vi "IR_UDP.vi"() -> ()   [LabVIEW 2015]
doc: "The myRIO Project template acquires acceleration data from the onboard accelerometer and displays the changes of acceleration values in a waveform chart."
uses:
  <vilib>/myRIO/Instrument Drivers/Utilities/Utilities.lvlib
  <vilib>/NIOSC/NI_OSC.lvlib
  <vilib>/NIOSC/Create Int32 Argument.vi
  <vilib>/NIOSC/Create Message_Single Arg.vi
  <vilib>/ptbypt/NI_PtbyPt.lvlib
  <vilib>/myRIO/Express VI/Onboard IO/AI/AI Express VI.xnode
  <vilib>/myRIO/Instrument Drivers/Onboard IO/AI/vis/Read.vi
  <vilib>/myRIO/Instrument Drivers/Onboard IO/AI/AI.lvlib
  <vilib>/myRIO/Common/Instrument Driver Framework/Utilities/typedefs/Analog Scaling Constants.ctl
  <vilib>/myRIO/Common/Instrument Driver Framework/Utilities/typedefs/Analog Scaling Constants List.ctl
  <vilib>/myRIO/Common/Instrument Driver Framework/myRIO v1.0/AI/typedefs/AI Channels Enum.ctl
  <vilib>/myRIO/Common/Instrument Driver Framework/myRIO v1.0/AI/typedefs/AI Channels List.ctl
  <vilib>/myRIO/Common/Instrument Driver Framework/Utilities/typedefs/Generic FPGA Reference.ctl
  <vilib>/myRIO/Common/Instrument Driver Framework/Utilities/typedefs/myRIO v1.0 Reference.ctl
  <vilib>/myRIO/Common/Instrument Driver Framework/Utilities/typedefs/Hardware Version Enum.ctl
  <vilib>/myRIO/Common/Instrument Driver Framework/Utilities/typedefs/myRIO Generic Hardware Reference.ctl
  <vilib>/myRIO/Instrument Drivers/Onboard IO/AI/typedefs/AI Reference.ctl
  <vilib>/myRIO/Instrument Drivers/Onboard IO/AI/vis/myRIO AI Open.xnode
  <vilib>/myRIO/Common/Instrument Driver Framework/Utilities/vis/Is FPGA Ref Available.vi
  <vilib>/myRIO/Common/Instrument Driver Framework/myRIO v1.0/AI/vis/myRIO v1.1 Open AI.vi
  <vilib>/userdefined/High Color/nirio_resource_hc.ctl
panel:
  out "numeric 2":dbl format="%_3g"
  in  "Koffset [cm] 2":dbl
  in  "Kscale [cm-V] 2":dbl=27.5
  out "Vo [V] 2":dbl format="%.2f"
  out "Range [cm] 2":dbl(knob) scale=0.0..10.0
  out "error out":errorcluster
  in  "Stop":bool
  # "Overview: The myRIO Project template acquires acceleration data from the onboard accelerometer and displays the changes of acceleration values in a waveform chart.\nInstructions:\n1. Check the myRIO target IP address in the project and make sure the target IP address is correct. \n2. Run this VI."
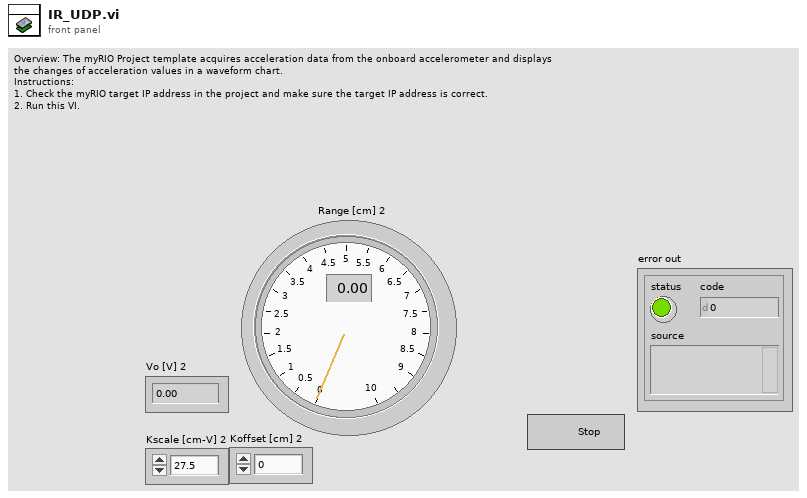
[diagram p1: front panel]
types:
  T1 = typedef "AI.lvlib/AI Reference.ctl" = cluster{"myRIO Reference":T2, "AI Channels List":T6, "AI Scaling Constants List":T8}
  T2 = typedef "myRIO Generic Hardware Reference.ctl" = cluster{"myRIO Model":T3, "myRIO Hardware Reference":T4}
  T3 = typedef "Hardware Version Enum.ctl" = enum16{"Unknown", "myRIO-1900", "myRIO-1950", "roboRIO"}
  T4 = typedef "myRIO v1.0 Reference.ctl" = cluster{"Generic FPGA Reference":T5, "Allow multiple opens":bool}
  T5 = typedef "Generic FPGA Reference.ctl" = refnum<k20>
  T6 = typedef "AI Channels List.ctl" = T7[]
  T7 = typedef "AI Channels Enum.ctl" = enum16{"Not Connected", "AudioIn/Left", "AudioIn/Right", "C/AI0", "C/AI1", "A/AI0", "A/AI1", "A/AI2", "A/AI3", "B/AI0", "B/AI1", "B/AI2", "B/AI3", "AI/AI0", "AI/AI1", "AI/AI2", "AI/AI3"}
  T8 = typedef "Analog Scaling Constants List.ctl" = T9[]
  T9 = typedef "Analog Scaling Constants.ctl" = cluster{"LSB Weight (Volts)":dbl, "Offset (Volts)":dbl, "Signed?":bool}
  T10 = typedef "nirio_resource_hc.ctl" = tag
  T11 = typedef "NI_OSC.lvlib/Argument.ctl" = cluster{"argument":string, "type tag":string}
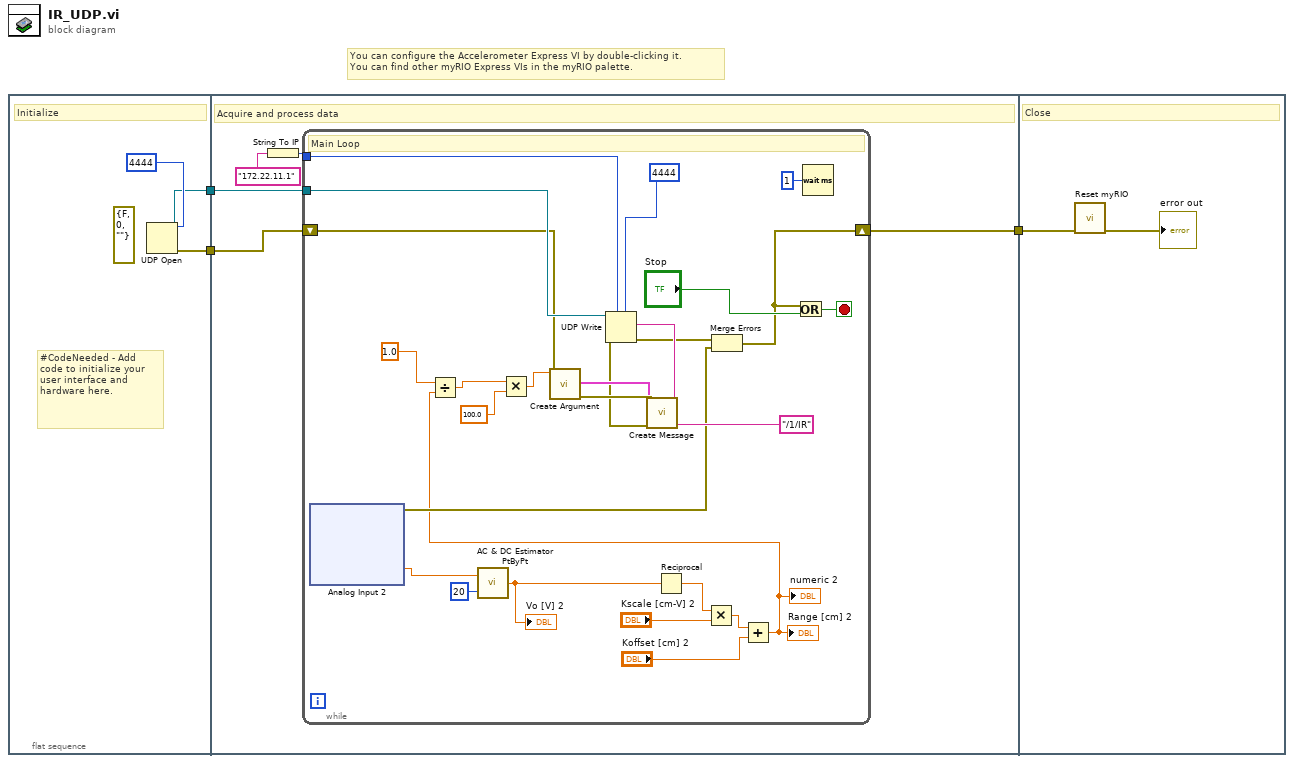
[diagram p0: block diagram]
diagram:
  # "You can configure the Accelerometer Express VI by double-clicking it.\nYou can find other myRIO Express VIs in the myRIO palette."
  n1 = flat-sequence {
    tunnel: [w4] -> w3
    tunnel: [w5] -> w2
    tunnel: w3 -> [w11]
    tunnel: w2 -> [w10]
    tunnel: [w7] -> w1
    tunnel: w1 -> [w76]
    frame #0 {
      (unwired) errorcluster {"status"=FALSE, "code"=0, "source"=""} ("error in (no error)")
      # "#CodeNeeded - Add code to initialize your user interface and hardware here."
      # "Initialize"
      n2 = UDP Open(11:u16 4444 ("port")) -> (port=w5:refnum<k16>, 0:w4:errorcluster)  [unwired: 4 in, 1 out]
    }
    frame #1 {
      # "Acquire and process data"
      n3 = String To IP(1:"172.22.11.1" ("data")) -> (0:w8:u32)
      n4 = while {
        shift-right: [w19] -> w7
        shift-left: w11 -> [w31]
        tunnel: w10 -> [w35]
        tunnel: w8 -> [w33]
        stop <- w37 stop-if-true
        # "Main Loop"
        n5 = xnode "Analog Input 2"() -> ("B/AI0 (Pin 3)"=w20:dbl, "error out"=w17:errorcluster)  [unwired: 1 in]
        n6 = call <vilib>:"AC & DC Estimator PtByPt.vi"("signal"=w20, "sample length"=20) -> ("DC estimate (V)"=w24:dbl)  [unwired: 1 in, 2 out]
        "Vo [V] 2" <- w24
        n7 = Reciprocal(x=w24) -> (1/x=w26:dbl)
        n8 = Multiply(x=w26, y="Kscale [cm-V] 2") -> (x*y=w21:dbl)
        n9 = Add(x=w21, y="Koffset [cm] 2") -> (x+y=w15:dbl)
        "Range [cm] 2" <- w15
        "numeric 2" <- w15
        n10 = Divide(x=1.0, y=w15) -> (x/y=w13:dbl)
        n11 = Multiply(x=w13, y=100.0) -> (x*y=w12:dbl)
        n12 = call-poly <vilib>:"Create Argument.vi"("error in"=w31, "int32 data"=w12) -> ("error out"=w30:errorcluster, "int32 argument"=w29:T11)  [unwired: 8 in]
        n13 = call-poly <vilib>:"Create Message.vi"("error in"=w30, "argument"=w29, "address pattern"="/1/IR") -> ("error out"=w28:errorcluster, "message"=w27:string)  [unwired: 7 in]
        n14 = UDP Write(address=w33, port or service name=u16 4444 ("port"), connection ID=w35, data in=w27, 8:w28) -> (error out=w18:errorcluster)  [unwired: 1 in, 1 out]
        n15 = Merge Errors(w18, w17) -> (w19:errorcluster)
        n16 = Or(x=w19, y="Stop") -> (x .or. y?=w37:bool)
        n17 = Wait (ms)(milliseconds to wait=u32 1) -> ()  [unwired: 1 out]
      }
    }
    frame #2 {
      # "Close"
      n18 = call <vilib>:"Reset myRIO.vi"("error in (no error)"=w76) -> ("error out"=→"error out":errorcluster)  [unwired: 10 in]
    }
  }
